vi "RichToFlatni_measurementlink_sessionmanagement_v1_RegisterMultiplexerSessionsRequest.vi"(5 "OutputClusterType":T1, 11 "InputCluster":T4) -> (3 "OutputCluster":T1)   [LabVIEW 2020, in "ni.measurementlink.sessionmanagement.v1.lvlib"]
uses:
  ni.measurementlink.sessionmanagement.v1.lvlib
  nidevice_grpc_Session_Flat.ctl
  ni_measurementlink_sessionmanagement_v1_MultiplexerSessionInformation_Flat.ctl
  ni_measurementlink_sessionmanagement_v1_RegisterMultiplexerSessionsRequest_Flat.ctl
  nidevice_grpc_Session.ctl
  ni_measurementlink_sessionmanagement_v1_MultiplexerSessionInformation.ctl
  ni_measurementlink_sessionmanagement_v1_RegisterMultiplexerSessionsRequest.ctl
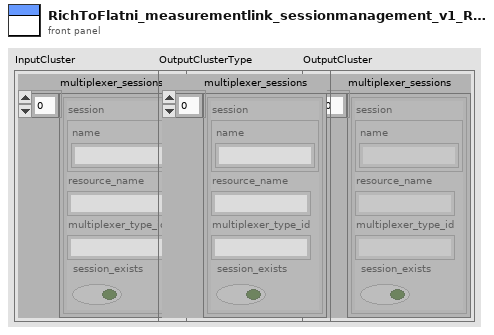
[diagram p1: front panel]
types:
  T1 = typedef "ni.measurementlink.sessionmanagement.v1.lvlib/ni_measurementlink_sessionmanagement_v1_RegisterMultiplexerSessionsRequest_Flat.ctl" = cluster{"multiplexer_sessions":T2[]}
  T2 = typedef "ni.measurementlink.sessionmanagement.v1.lvlib/ni_measurementlink_sessionmanagement_v1_MultiplexerSessionInformation_Flat.ctl" = cluster{"session":T3, "resource_name":string, "multiplexer_type_id":string, "session_exists":bool}
  T3 = typedef "ni.measurementlink.sessionmanagement.v1.lvlib/nidevice_grpc_Session_Flat.ctl" = cluster{"name":string}
  T4 = typedef "ni.measurementlink.sessionmanagement.v1.lvlib/ni_measurementlink_sessionmanagement_v1_RegisterMultiplexerSessionsRequest.ctl" = cluster{"multiplexer_sessions":T5[]}
  T5 = typedef "ni.measurementlink.sessionmanagement.v1.lvlib/ni_measurementlink_sessionmanagement_v1_MultiplexerSessionInformation.ctl" = cluster{"session":T6, "resource_name":string, "multiplexer_type_id":string, "session_exists":bool}
  T6 = typedef "ni.measurementlink.sessionmanagement.v1.lvlib/nidevice_grpc_Session.ctl" = cluster{"name":string}
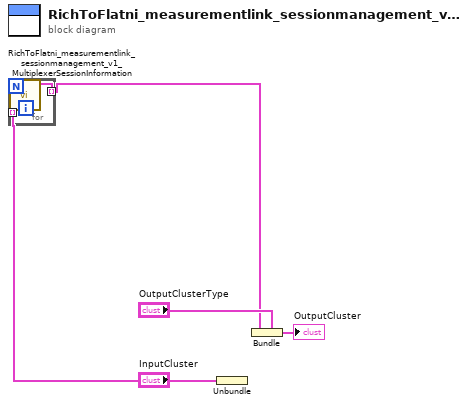
[diagram p0: block diagram]
diagram:
  n1 = Unbundle "Unbundle"("InputCluster") -> ("multiplexer_sessions"=w2:T5[])
  n2 = for {
    tunnel: w2 -> [w7] mode=indexing
    tunnel: [w6] -> w1 mode=indexing
    n3 = call "RichToFlatni_measurementlink_sessionmanagement_v1_MultiplexerSessionInformation.vi"("InputCluster"=w7) -> ("OutputCluster"=w6:T2)  [unwired: 10 in]
  }
  n4 = Bundle "Bundle"(cluster="OutputClusterType", "multiplexer_sessions"=w1) -> (→"OutputCluster":T1)
